vi "Ready_measurement.vi"() -> ()   [LabVIEW 2024]
uses:
  <vilib>/Instr/_visa.llb/VISA Configure Serial Port (Instr).vi
  support/Serial - ASCII Characters.ctl
  support/Serial - XON-XOFF Characters.ctl
  support/Serial - Settings.ctl
panel:
  in  "Measure?":bool
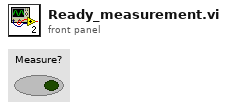
[diagram p1: front panel]
types:
  T1 = typedef "Serial - Settings.ctl" = cluster{"baud rate":u32, "data bits":u16, "parity":enum16{"None", "Odd", "Even", "Mark", "Space"}, "stop bits":u16, "flow control":u16}
  T2 = typedef "Serial - XON-XOFF Characters.ctl" = cluster{"XON":T3, "XOFF":T3}
  T3 = typedef "Serial - ASCII Characters.ctl" = enum16{"NUL", "SOH", "STX", "ETX", "EOT", "ENQ", "ACK", "BEL", "BS", "HT", "LF", "VT", "FF", "CR", "SO", "SI", "DLE", "DC1", "DC2", "DC3", "DC4", "NAK", "SYN", "ETB", "CAN", "EM", "SUB", "ESC", "FS", "GS", "RS", "US", "SP", "!", "\"", "#", "$", "%", "&", "'", "(", ")", "*", "+", ",", "- (-)", ".", "/", "0", "1", "2", "3", "4", "5", "6", "7", "8", "9", ":", ";", "<", "=", ">", "?", "@", "A", "B", "C", "D", "E", "F", "G", "H", "I", "J", "K", "L", "M", "N", "O", "P", "Q", "R", "S", "T", "U", "V", "W", "X", "Y", "Z", "[", "\\", "]", "^", "_", "`", "a", "b", "c", "d", "e", "f", "g", "h", "i", "j", "k", "l", "m", "n", "o", "p", "q", "r", "s", "t", "u", "v", "w", "x", "y", "z", "{", "|", "}", "~"}
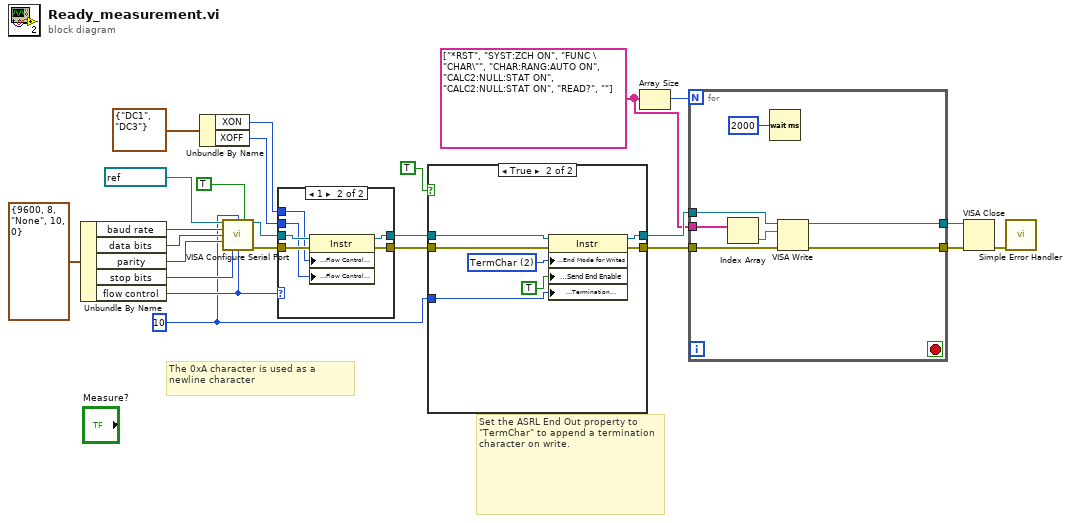
[diagram p0: block diagram]
diagram:
  w1 = string[] ["*RST", "SYST:ZCH ON", "FUNC \"CHAR\"", "CHAR:RANG:AUTO ON", "CALC2:NULL:STAT ON", "CALC2:NULL:STAT ON", "READ?", ""] ("Commands")
  w3 = u8 10 ("Termination Character")
  # "The 0xA character is used as a newline character"
  # "Set the ASRL End Out property to \"TermChar\" to append a termination character on write."
  n1 = Unbundle By Name(T1 {"baud rate"=9600, "data bits"=8, "parity"=enum."None", "stop bits"=10, "flow control"=0} ("Serial Settings")) -> ("baud rate"=w17:u32, "data bits"=w18:u16, "parity"=w19:enum16{"None", "Odd", "Even", "Mark", "Space"}, "stop bits"=w20:u16, "flow control"=w11:u16)
  n2 = Unbundle By Name(T2 {"XON"=enum."DC1", "XOFF"=enum."DC3"} ("XON/XOFF Characters")) -> ("XON"=w10:T3, "XOFF"=w9:T3)
  n3 = call-poly "VISA Configure Serial Port"("VISA resource name"=refnum<visa-resource-name> "COM1", "termination char\n(0xA = '\\n' = LF)"=w3, "Enable Termination\nChar (T)"=TRUE ("End Read on Termination Character?"), "baud rate (9600)"=w17, "data bits (8)"=w18, "parity (0:none)"=w19, "stop bits (10: 1 bit)"=w20, "flow control (0:none)"=w11) -> ("VISA resource name out"=w21:refnum<visa-resource-name>, "error out"=w22:errorcluster)  [unwired: 2 in, 4 out]
  n4 = case shown="1" w11 {
    tunnel: [w25 w32] -> w8
    tunnel: [w26 w31] -> w6
    tunnel: w22 -> [w25 w30]
    tunnel: w21 -> [w26 w29]
    tunnel: w10 -> [_ w28]
    tunnel: w9 -> [_ w27]
    frame Default {
    }
    frame 1 {
      n5 = property class="Instr"(reference=w29, error in=w30, "Serial Settings:Flow Control XON Character"=w28, "Serial Settings:Flow Control XOFF Character"=w27) -> (reference out=w31:refnum<visa-resource-name>, error out=w32:errorcluster)
    }
  }
  n6 = case shown="True" TRUE ("End Write on Termination Character?") {
    tunnel: w6 -> [w33 w41]
    tunnel: w8 -> [w34 w40]
    tunnel: [w33 w39] -> w5
    tunnel: [w34 w38] -> w7
    tunnel: w3 -> [_ w36]
    frame False {
    }
    frame True {
      w37 = u16 2 items=["None", "LastBit", "TermChar", "Break"] ("Serial Settings:Serial End Mode for Writes")
      n7 = property class="Instr"(reference=w41, error in=w40, "Serial Settings:End Mode for Writes"=w37, "Message Based Settings:Send End Enable"=TRUE, "Message Based Settings:Termination Character"=w36) -> (reference out=w39:refnum<visa-resource-name>, error out=w38:errorcluster)
    }
  }
  n8 = Array Size(array=w1) -> (size(s)=w2:i32)
  n9 = for {
    N: w2 -> [_]
    tunnel: w1 -> [w48]
    tunnel: w5 -> [w47]
    tunnel: w7 -> [w44]
    tunnel: [w42] -> w12
    tunnel: [w43] -> w13
    stop <- _ stop-if-true
    n10 = Index Array(array=w48) -> (element=w45:string)  [unwired: 1 in]
    n11 = Wait (ms)(milliseconds to wait=u32 2000) -> ()  [unwired: 1 out]
    n12 = VISA Write(VISA resource name=w47, write buffer=w45, error in (no error)=w44) -> (VISA resource name out=w42:refnum<visa-resource-name>, error out=w43:errorcluster)  [unwired: 1 out]
  }
  n13 = VISA Close(VISA resource name=w12, error in (no error)=w13) -> (error out=w14:errorcluster)
  n14 = call <vilib>:"Simple Error Handler.vi"("error in (no error)"=w14) -> ()  [unwired: 1 in, 8 out]
